vi "getting_started.vi"() -> ()   [LabVIEW 2015]
panel:
  in  "stop":bool
  out "Waveform Chart":cluster{sgl, sgl, sgl, sgl}(graph)
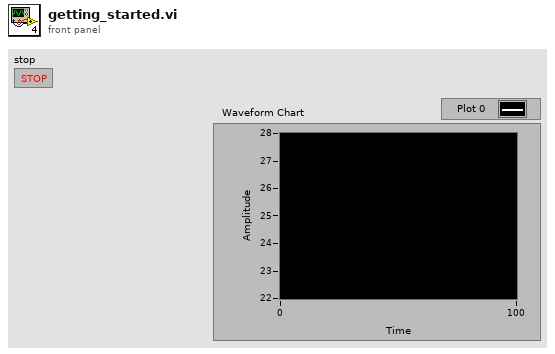
[diagram p1: front panel]
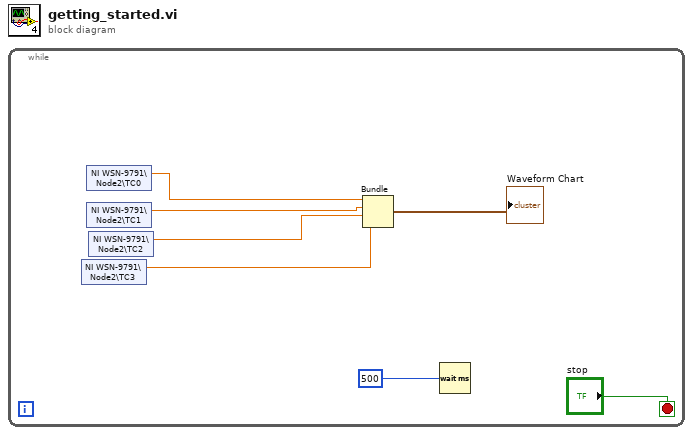
[diagram p0: block diagram]
diagram:
  n1 = while {
    stop <- "stop" stop-if-true
    n2 = shared-variable "NI WSN-9791\\Node2\\TC3"() -> (w3:sgl)  [unwired: 1 in, 1 out]
    n3 = shared-variable "NI WSN-9791\\Node2\\TC0"() -> (w6:sgl)  [unwired: 1 in, 1 out]
    n4 = shared-variable "NI WSN-9791\\Node2\\TC1"() -> (w5:sgl)  [unwired: 1 in, 1 out]
    n5 = shared-variable "NI WSN-9791\\Node2\\TC2"() -> (w4:sgl)  [unwired: 1 in, 1 out]
    n6 = Bundle(w6, w5, w4, w3) -> (→"Waveform Chart":cluster{sgl, sgl, sgl, sgl})  [unwired: 1 in]
    n7 = Wait (ms)(milliseconds to wait=500) -> ()  [unwired: 1 out]
  }
